vi "Read Voltage.vi"(8 "error in (no error)":errorcluster, 11 "Multifunction IO in":refnum<class "Multifunction IO.lvclass">) -> (0 "error out":errorcluster, 2 "Status":string, 3 "Multifunction IO out":refnum<class "Multifunction IO.lvclass">)   [LabVIEW 2020, in "Multifunction IO.lvclass"]
uses:
  Multifunction IO.lvclass
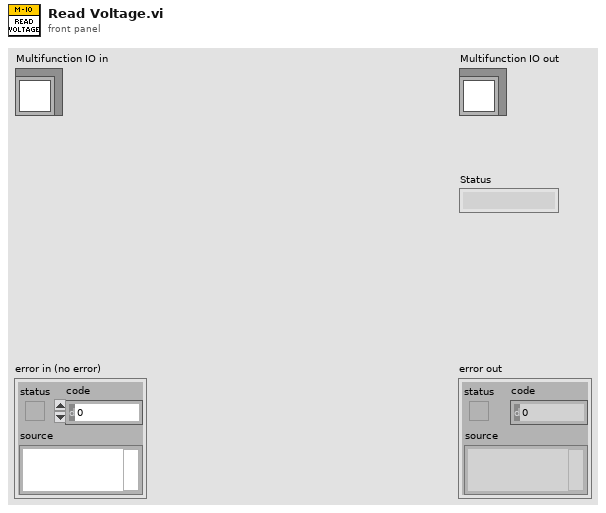
[diagram p1: front panel]
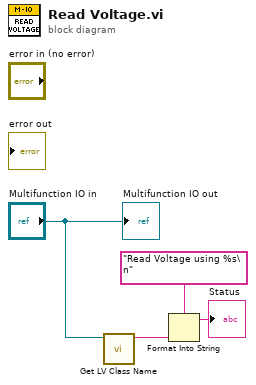
[diagram p0: block diagram]
diagram:
  n1 = call <vilib>:"Get LV Class Name.vi"("object"="Multifunction IO in") -> ("class name"=w4:string)  [unwired: 9 in, 1 out]
  n2 = Format Into String(format string="Read Voltage using %s\n", w4) -> (resulting string=→"Status":string)  [unwired: 2 in, 1 out]
  "Multifunction IO out" <- "Multifunction IO in"
